vi "GetDiagramLocals.vi"(5 "Diagram":refnum<class "Diagram.lvclass">, 6 "error in":errorcluster, 9 "VI Interpreter in":refnum<class "VI Interpreter.lvclass">) -> (0 "error out":errorcluster, 3 "VI Interpreter out":refnum<class "VI Interpreter.lvclass">, 4 "Diagram out":refnum<class "Diagram.lvclass">)   [LabVIEW 2014, in "VI Interpreter.lvclass"]
uses:
  VI Interpreter.lvclass
  Diagram/Diagram.lvclass
  Diagram/Diagram.lvclass/Diagram.ctl
  Local/Local.lvclass
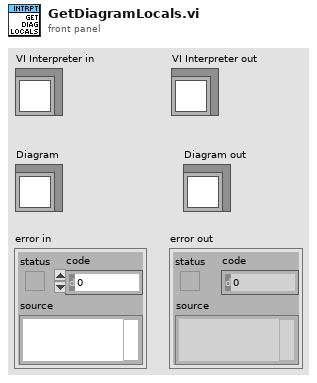
[diagram p1: front panel]
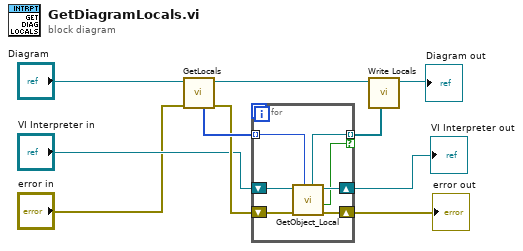
[diagram p0: block diagram]
diagram:
  n1 = call "GetLocals.vi"("error in"="error in", "Diagram in"="Diagram") -> ("error out"=w9:errorcluster, "Diagram out"=w2:refnum<class "Diagram.lvclass">, "locals"=w10:i32[])  [unwired: 5 in]
  n2 = for {
    shift-right: [w13] -> w8
    shift-left: "VI Interpreter in" -> [w17]
    tunnel: w10 -> [w16] mode=indexing
    shift-right: [w15] -> w7
    shift-left: w9 -> [w14]
    tunnel: [w12] -> w3 mode=indexing if=w11
    n3 = call "GetObject_Local.vi"("UID"=w16, "error in"=w14, "VI Interpreter in"=w17) -> ("error out"=w15:errorcluster, "found"=w11:bool, "VI Interpreter out"=w13:refnum<class "VI Interpreter.lvclass">, "local"=w12:refnum<class "Local.lvclass">)  [unwired: 3 in]
  }
  "error out" <- w7
  "VI Interpreter out" <- w8
  n4 = call "Write Locals.vi"("Locals"=w3, "Diagram in"=w2) -> ("Diagram out"=→"Diagram out":refnum<class "Diagram.lvclass">)  [unwired: 7 in]
